vi "LinDaten Datei open.vi"(11 "selected path (Eingang)":path) -> (0 "Fehler (Ausgang)":errorcluster, 3 "selected path (Ausgang)":path)   [LabVIEW 2020, in "Linearisierung v2.lvlib"]
uses:
  Linearisierung v2.lvlib
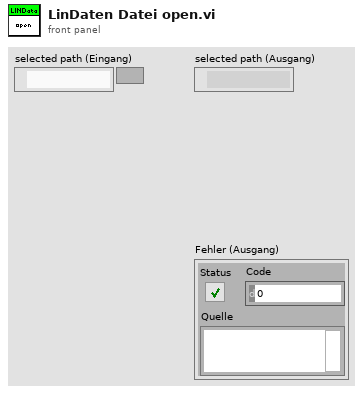
[diagram p1: front panel]
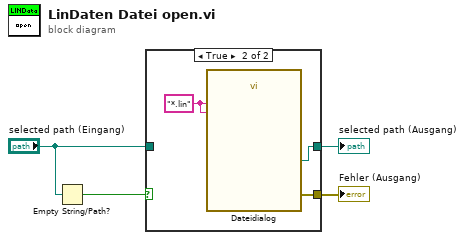
[diagram p0: block diagram]
diagram:
  n1 = Empty String/Path?(string/path="selected path (Eingang)") -> (empty?=w1:bool)
  n2 = case shown="True" w1 {
    tunnel: [w5 w8] -> w3
    tunnel: [_ w6] -> w4
    tunnel: "selected path (Eingang)" -> [w5 _]
    frame False {
    }
    frame True {
      w7 = "*.lin" ("pattern (all files)")
      n3 = call "Dateidialog"("pattern (all files)"=w7, "pattern label"=w7) -> ("selected path"=w8:path, "error out"=w6:errorcluster)  [unwired: 10 in, 2 out]
    }
  }
  "Fehler (Ausgang)" <- w4
  "selected path (Ausgang)" <- w3
